vi "Measure ADC Select.vi"(0 "VISA resource name":refnum<visa-resource-name>, 5 "Node In":string, 7 "Select ADC Type":u8(ring)=1 items=["Integrating ADC", "Fast ADC"], 11 "error in (no error)":errorcluster) -> (4 "VISA resource name out":refnum<visa-resource-name>, 6 "Node Out":string, 15 "error out":errorcluster)   [LabVIEW 2013, in "Keithley 2600 Series.lvlib"]
doc: "The SMU has two types of analog to digital converter for making measurements. This attribute controls which analog to digital converter to use. This feature is exclusive to the 265x line of instruments.\n\n<b>Functions and Attributes Used</b>\nsmux.measure.adc"
uses:
  Keithley 2600 Series.lvlib
  Private/GlobalVariables.vi
panel:
  # "(c) 2010 Keithley Instruments, Inc.  ALL RIGHTS RESERVED."
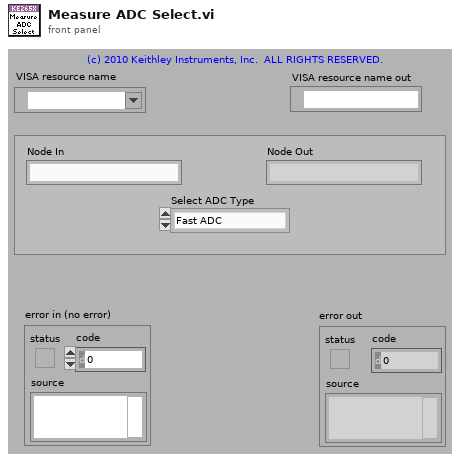
[diagram p1: front panel]
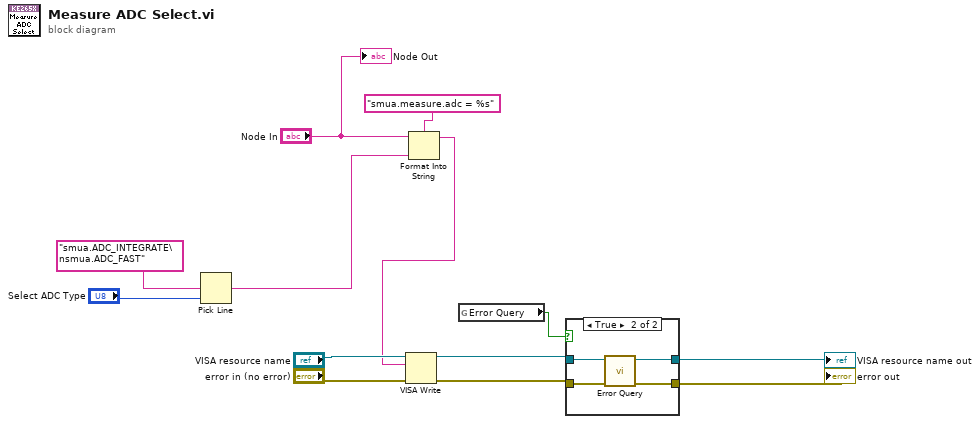
[diagram p0: block diagram]
diagram:
  n1 = Pick Line(multi-line string="smua.ADC_INTEGRATE\nsmua.ADC_FAST", line index="Select ADC Type") -> (output string=w6:string)  [unwired: 1 in]
  n2 = Format Into String(format string="smua.measure.adc = %s", initial string="Node In", w6) -> (resulting string=w1:string)  [unwired: 1 in, 1 out]
  n3 = VISA Write(VISA resource name="VISA resource name", write buffer=w1, error in (no error)="error in (no error)") -> (VISA resource name out=w5:refnum<visa-resource-name>, error out=w4:errorcluster)  [unwired: 1 out]
  n4 = global read "GlobalVariables.vi" "Error Query"() -> (w13:bool)
  n5 = case shown="True" w13 {
    tunnel: w5 -> [w15 w19]
    tunnel: w4 -> [w14 w18]
    tunnel: [w15 w17] -> w12
    tunnel: [w14 w16] -> w11
    frame False {
    }
    frame True {
      n6 = call "Error Query.vi"("error in (no error)"=w18, "VISA resource name"=w19) -> ("error out"=w16:errorcluster, "VISA resource name out"=w17:refnum<visa-resource-name>)  [unwired: 8 out]
    }
  }
  "VISA resource name out" <- w12
  "error out" <- w11
  "Node Out" <- "Node In"
